vi "Recurse.vi"(7 "Actor in":refnum<class "Actor.lvclass">, 10 "Msg":refnum<class "Msg.lvclass">) -> (0 "Error out":errorcluster, 2 "Msg Output":refnum<class "Msg Output.lvclass">, 5 "Actor out":refnum<class "Actor.lvclass">)   [LabVIEW 2025, in "jettl.lvlib"]
uses:
  jettl.lvlib
  Actor/Actor.lvclass
  Msg/Msg.lvclass
  Msg Output/Msg Output.lvclass
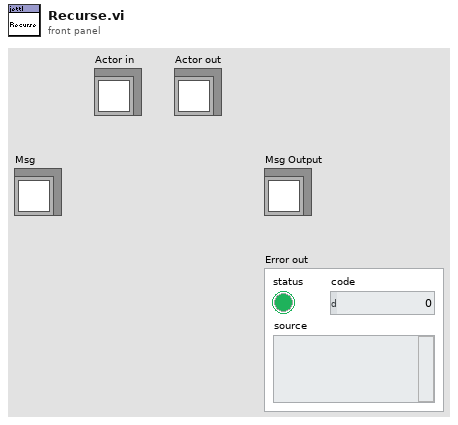
[diagram p1: front panel]
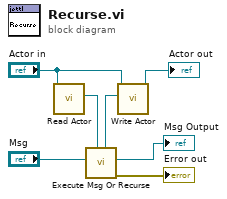
[diagram p0: block diagram]
diagram:
  n1 = call-dynamic "Read Actor.vi"("Actor in"="Actor in") -> ("Actor"=w2:refnum<class "Actor.lvclass">)  [unwired: 10 in]
  n2 = call "Execute Msg Or Recurse.vi"("Actor in"=w2, "Msg"="Msg") -> ("Error out"=→"Error out":errorcluster, "Msg Output"=→"Msg Output":refnum<class "Msg Output.lvclass">, "Actor out"=w3:refnum<class "Actor.lvclass">)  [unwired: 7 in]
  n3 = call-dynamic "Write Actor.vi"("Actor"=w3, "Actor in"="Actor in") -> ("Actor out"=→"Actor out":refnum<class "Actor.lvclass">)  [unwired: 9 in]
